vi "外观 2.vi"(0 "Data In":T4 caption="数据输入", 2 "Display State In":T2 caption="显示状态输入", 3 "Container State":T3 caption="容器状态") -> (6 "Data Out":T4 caption="数据输出", 7 "Display State Out":T2 caption="显示状态输出", 8 "Action":T1 caption="动作")   [LabVIEW 2016, in "水质测量数据.xctl"]
uses:
  <vilib>/_xctls/Container State.ctl
  <vilib>/_xctls/Action.ctl
  <vilib>/_xctls/XControlSupport.lvlib
panel:
  out "平行样数据标识":string
  out "平行样实测值":string
  out "平行样数据时间":string
  out "加标回收数据标识":string
  out "加标回收实测值":string
  out "加标回收数据时间":string
  out "跨度核查数据标识":string
  out "跨度核查实测值":string
  out "跨度核查数据时间":string
  out "零点核查数据标识":string
  out "零点核查实测值":string
  out "零点核查数据时间":string
  out "空白数据标识":string
  out "空白实测值":string
  out "空白数据时间":string
  out "标样数据标识":string
  out "标样实测值":string
  out "标样数据时间":string
  out "因子编码":string
  out "水样数据标识":string
  out "水样实测值":string
  out "水样数据时间":string
  out "标样参考值":string
  out "单位":string
  # "因子编码:"
  # "零点核查数据时间:"
  # "单位:"
  # "零点核查实测值:"
  # "标样参考值:"
  # "零点核查数据标识:"
  # "水样数据时间:"
  # "跨度核查数据时间:"
  # "水样实测值:"
  # "跨度核查实测值:"
  # "水样数据标识:"
  # "跨度核查数据标识:"
  # "标样数据时间:"
  # "加标回收数据时间:"
  # "标样实测值:"
  # "加标回收实测值:"
  # "标样数据标识:"
  # "加标回收数据标识:"
  # "空白数据时间:"
  # "平行样数据时间:"
  # "空白实测值:"
  # "平行样实测值:"
  # "空白数据标识:"
  # "平行样数据标识:"
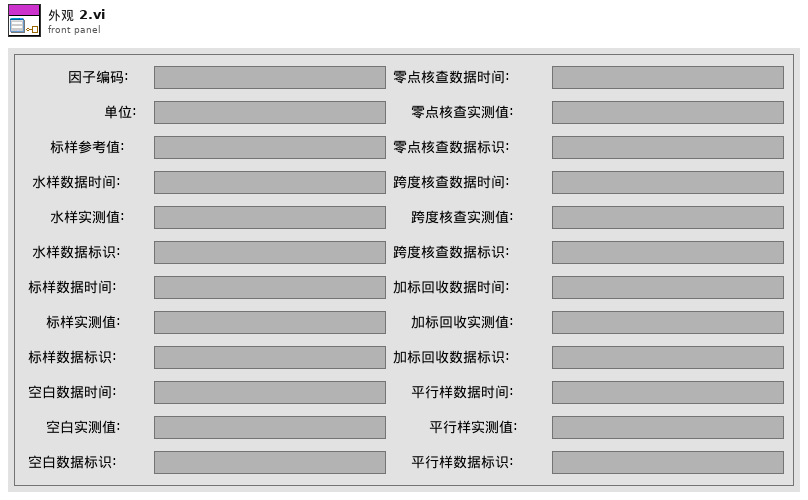
[diagram p1: front panel]
types:
  T1 = typedef "XControlSupport.lvlib/Action.ctl" = cluster{"Data Changed?":bool, "State Changed?":bool, "Action Name":string}
  T2 = typedef "水质测量数据.xctl/状态 2.ctl" = cluster{"Numeric":dbl}
  T3 = typedef "XControlSupport.lvlib/Container State.ctl" = cluster{"Indicator?":bool, "Run Mode?":bool, " Refnum":refnum<vi>}
  T4 = typedef "水质测量数据.xctl/数据 2.ctl" = cluster{"单位":string, "标样参考值":string, "水样数据时间":string, "水样实测值":string, "水样数据标识":string, "因子编码":string, "标样数据时间":string, "标样实测值":string, "标样数据标识":string, "空白数据时间":string, "空白实测值":string, "空白数据标识":string, "零点核查数据时间":string, "零点核查实测值":string, "零点核查数据标识":string, "跨度核查数据时间":string, "跨度核查实测值":string, "跨度核查数据标识":string, "加标回收数据时间":string, "加标回收实测值":string, "加标回收数据标识":string, "平行样数据时间":string, "平行样实测值":string, "平行样数据标识":string}
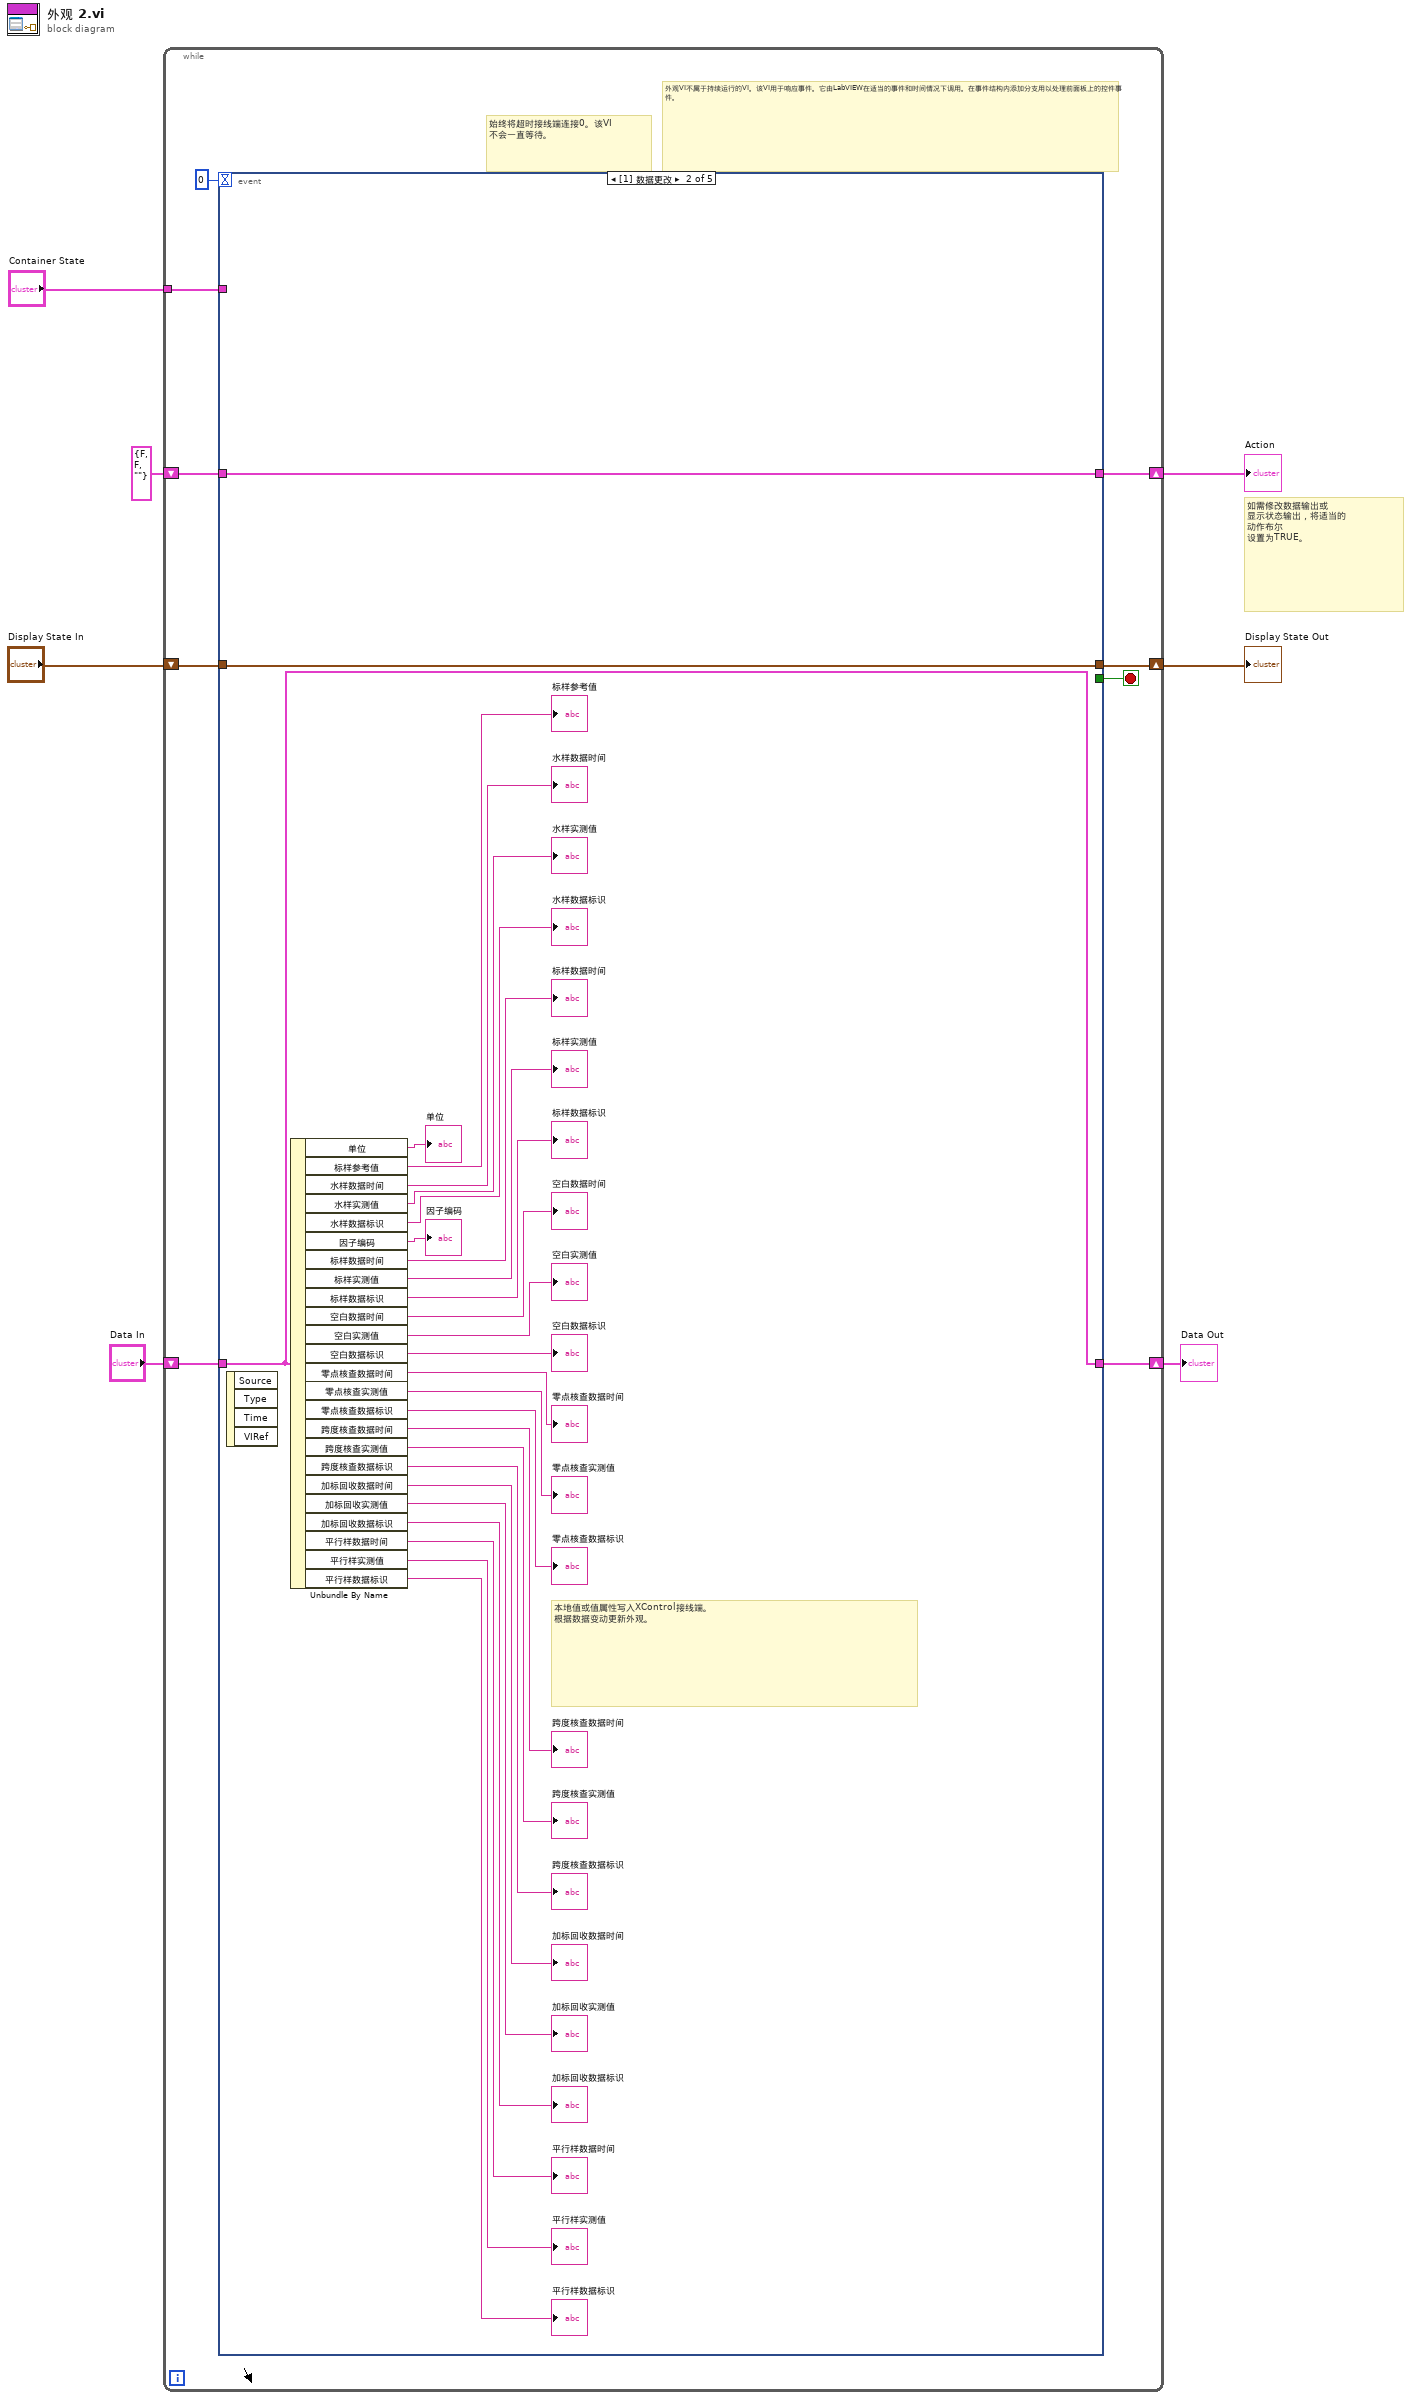
[diagram p0: block diagram]
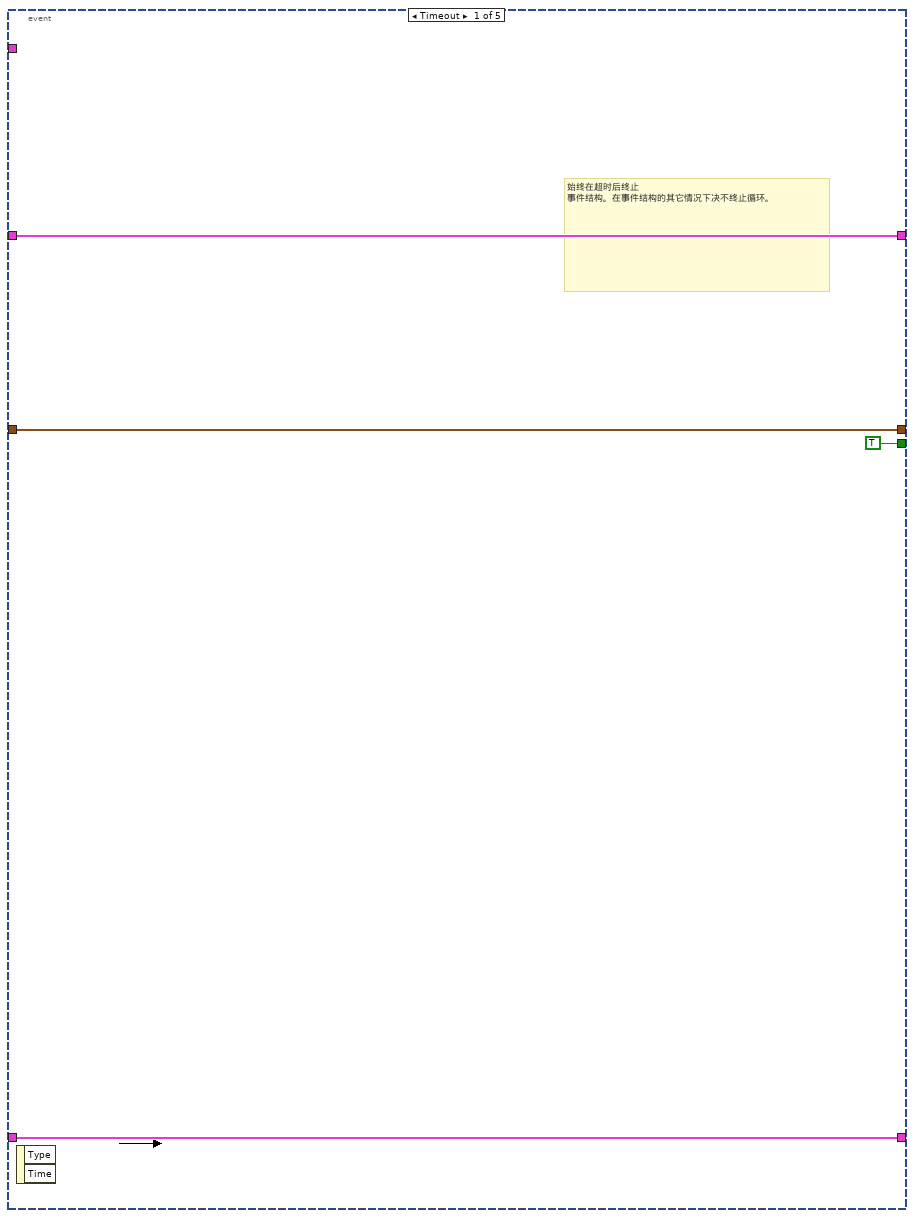
[diagram p2: hidden frame]
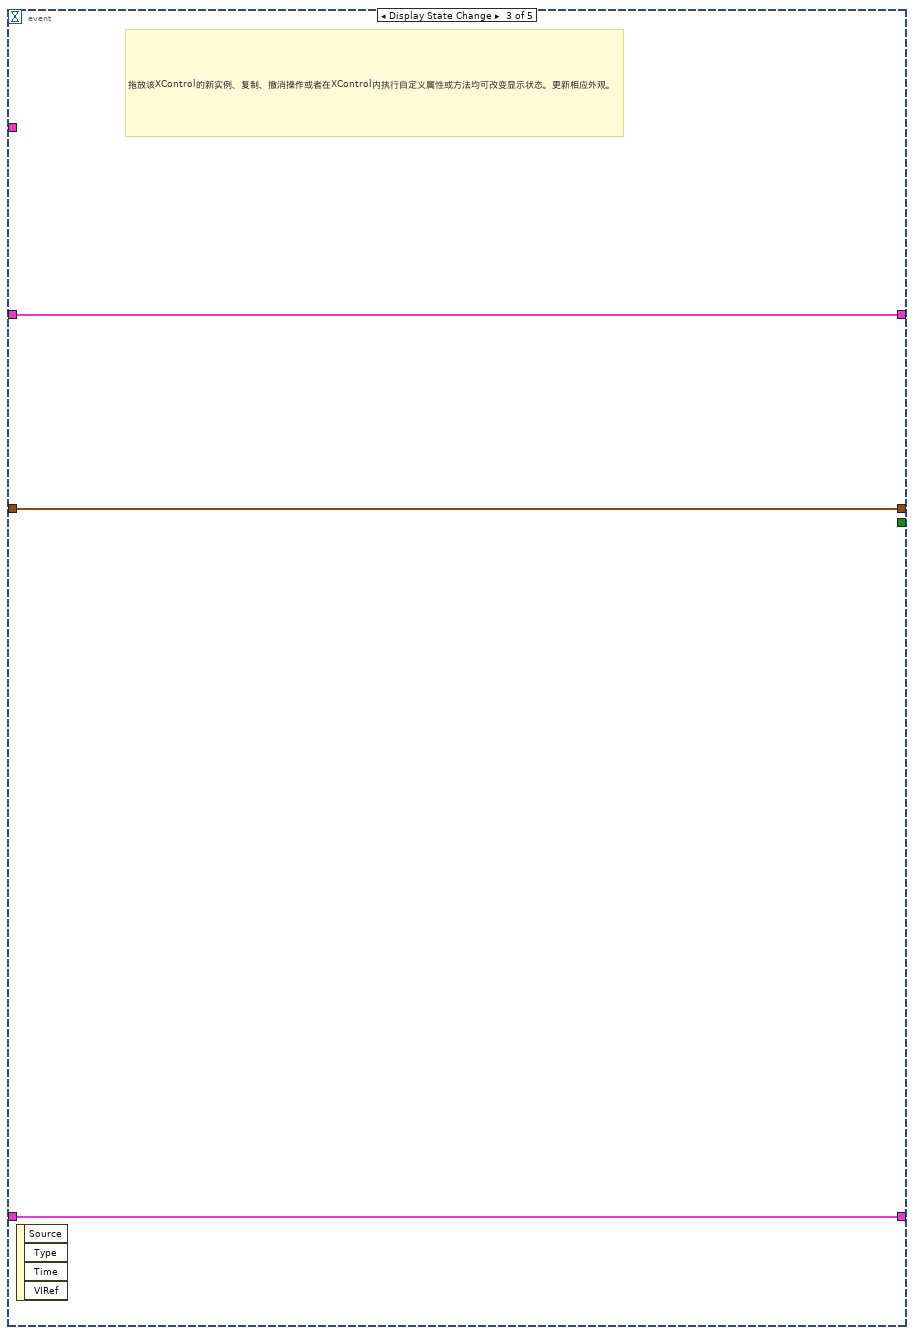
[diagram p3: hidden frame]
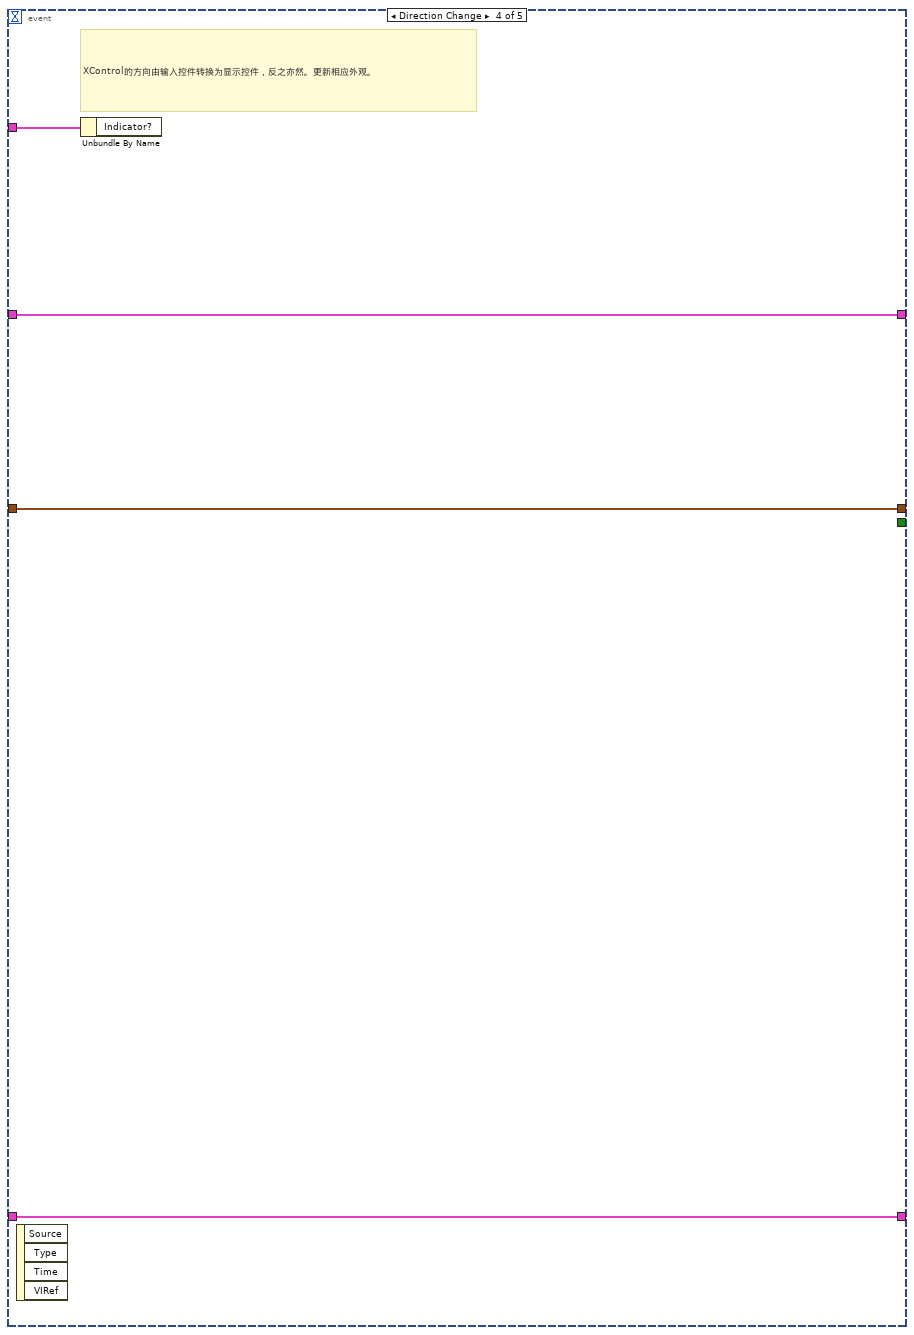
[diagram p4: hidden frame]
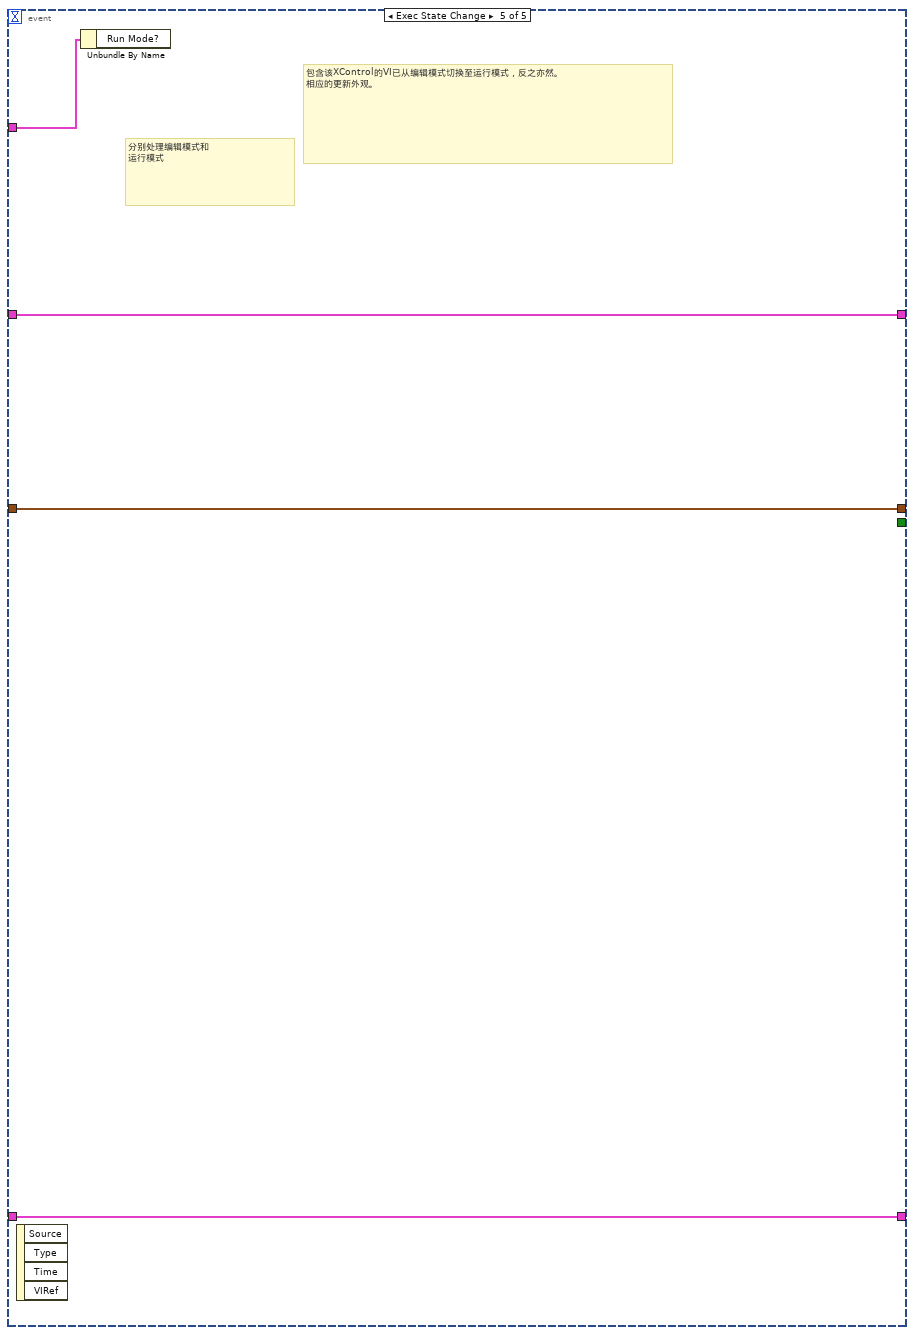
[diagram p5: hidden frame]
diagram:
  # "如需修改数据输出或\n显示状态输出，将适当的\n动作布尔\n设置为TRUE。"
  n1 = while {
    shift-right: [w15] -> w4
    shift-left: "Display State In" -> [w16]
    tunnel: "Container State" -> [w12]
    shift-right: [w10] -> w7
    shift-left: "Data In" -> [w11]
    shift-right: [w8] -> w2
    shift-left: T1 {"Data Changed?"=FALSE, "State Changed?"=FALSE, "Action Name"=""} ("Action") -> [w9]
    stop <- w14 stop-if-true
    # "外观VI不属于持续运行的VI。该VI用于响应事件。它由LabVIEW在适当的事件和时间情况下调用。在事件结构内添加分支用以处理前面板上的控件事件。"
    # "始终将超时接线端连接0。该VI\n不会一直等待。"
    n2 = event shown="[1] 数据更改" {
      selector: _ -> [_ _ _ _ _]
      dyn-events: _ -> [_ _ _ _ _]
      timeout: 0 -> [_ _ _ _ _]
      tunnel: w16 -> [w18 w46 w50 w53 w57]
      tunnel: [w18 w46 w50 w53 w57] -> w15
      tunnel: [TRUE _ _ _ _] -> w14
      tunnel: w12 -> [_ _ _ w54 w58]
      tunnel: w11 -> [w17 w45 w49 w52 w56]
      tunnel: [w17 w45 w49 w52 w56] -> w10
      tunnel: [w19 w47 w48 w51 w55] -> w8
      tunnel: w9 -> [w19 w47 w48 w51 w55]
      event Timeout {
        # "始终在超时后终止\n事件结构。在事件结构的其它情况下决不终止循环。"
        n3 = event-data() -> ()  [unwired: 1 in, 2 out]
      }
      event Data Change {
        # "本地值或值属性写入XControl接线端。\n根据数据变动更新外观。"
        n4 = event-data() -> ()  [unwired: 1 in, 4 out]
        n5 = Unbundle By Name(w45) -> ("单位"=→"单位":string, "标样参考值"=→"标样参考值":string, "水样数据时间"=→"水样数据时间":string, "水样实测值"=→"水样实测值":string, "水样数据标识"=→"水样数据标识":string, "因子编码"=→"因子编码":string, "标样数据时间"=→"标样数据时间":string, "标样实测值"=→"标样实测值":string, "标样数据标识"=→"标样数据标识":string, "空白数据时间"=→"空白数据时间":string, "空白实测值"=→"空白实测值":string, "空白数据标识"=→"空白数据标识":string, "零点核查数据时间"=→"零点核查数据时间":string, "零点核查实测值"=→"零点核查实测值":string, "零点核查数据标识"=→"零点核查数据标识":string, "跨度核查数据时间"=→"跨度核查数据时间":string, "跨度核查实测值"=→"跨度核查实测值":string, "跨度核查数据标识"=→"跨度核查数据标识":string, "加标回收数据时间"=→"加标回收数据时间":string, "加标回收实测值"=→"加标回收实测值":string, "加标回收数据标识"=→"加标回收数据标识":string, "平行样数据时间"=→"平行样数据时间":string, "平行样实测值"=→"平行样实测值":string, "平行样数据标识"=→"平行样数据标识":string)
      }
      event Display State Change {
        # "拖放该XControl的新实例、复制、撤消操作或者在XControl内执行自定义属性或方法均可改变显示状态。更新相应外观。"
        n6 = event-data() -> ()  [unwired: 1 in, 4 out]
      }
      event Direction Change {
        # "XControl的方向由输入控件转换为显示控件，反之亦然。更新相应外观。"
        n7 = event-data() -> ()  [unwired: 1 in, 4 out]
        n8 = Unbundle By Name(w54) -> ()  [unwired: 1 out]
      }
      event Exec State Change {
        # "包含该XControl的VI已从编辑模式切换至运行模式，反之亦然。\n相应的更新外观。"
        # "分别处理编辑模式和\n运行模式"
        n9 = event-data() -> ()  [unwired: 1 in, 4 out]
        n10 = Unbundle By Name(w58) -> ()  [unwired: 1 out]
      }
    }
  }
  "Display State Out" <- w4
  "Data Out" <- w7
  "Action" <- w2
